vi "平行样数据插入.vi"(8 "error in (no error)":errorcluster, 11 "平行样测试数据":T1={"时间"=timestamp(0 s since 1904-01-01), "参数"="", "数据类型"="N", "第一次水样浓度值"=0.0, "第二次水样测试时间"=timestamp(0 s since 1904-01-01), "第二次水样浓度值"=0.0}) -> (0 "error out":errorcluster)   [LabVIEW 2016, in "质控单元V1.lvlib"]
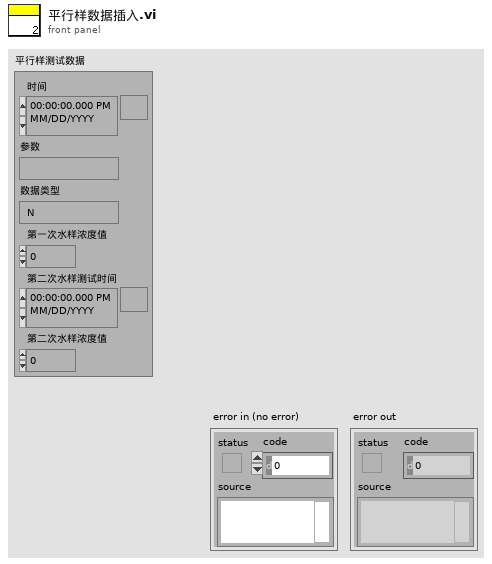
[diagram p1: front panel]
types:
  T1 = typedef "平行样测试数据字段定义.ctl" = cluster{"时间":timestamp, "参数":string, "数据类型":string, "第一次水样浓度值":dbl, "第二次水样测试时间":timestamp, "第二次水样浓度值":dbl}
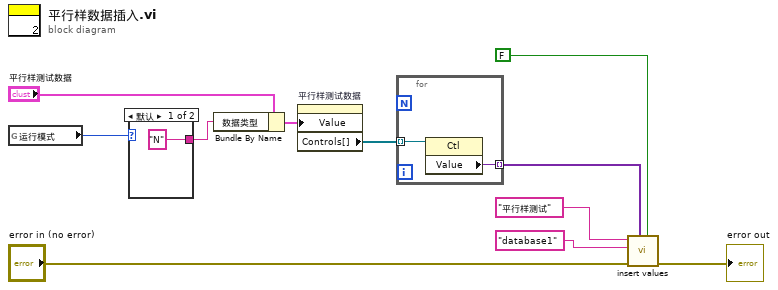
[diagram p0: block diagram]
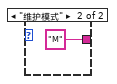
[diagram p2: hidden frame]
diagram:
  n1 = global read "系统交互.vi" "运行模式"() -> (w11:enum16{"维护模式", "常规模式", "应急模式", "质控模式"})
  n2 = case shown="默认" w11 {
    tunnel: ["N" "M"] -> w10
    frame Default {
    }
    frame "维护模式" {
    }
  }
  n3 = Bundle By Name(cluster="平行样测试数据", "数据类型"=w10) -> (w2:T1)
  n4 = property on="平行样测试数据" class="Clust (严格)"("Value"=w2) -> ("Controls[]"=w1:refnum<vi>[])  [unwired: 2 in, 2 out]
  n5 = for {
    tunnel: [w15] -> w5 mode=indexing
    tunnel: w1 -> [w14] mode=indexing
    n6 = property class="Ctl"(reference=w14) -> ("Value"=w15:variant)  [unwired: 1 in, 2 out]
  }
  n7 = call "insert values.vi"("是否创建唯一键"=FALSE, "data"=w5, "错误输入（无错误）"="error in (no error)", "database"="database1", "Tabe Name"="平行样测试" ("table")) -> ("错误输出"=→"error out":errorcluster)  [unwired: 6 in]
